vi "Periodic Tasks.vi"(8 "error in":errorcluster) -> ()   [LabVIEW 2017]
doc: "This VI runs in parallel to other tasks. It can contain as many user-defined periodic loops as you need. These can carry out PID or other sorts of timed response."
uses:
  elevator_control.ctl
  Intake_control.ctl
  <vilib>/Rock Robotics/WPI/ThirdParty/Phoenix-LabVIEW/Motor Controller/Controls/CTRE_Phoenix_MotorControl_ControlMode.ctl
  <vilib>/Rock Robotics/WPI/DriverStation/WPI_DriverStationRobotMode2.ctl
  <vilib>/Rock Robotics/WPI/Solenoid/WPI_SolenoidValue.ctl
  LabVIEW_is_Under_Control.lib/Util/Toggle/Change Detect.vi
  LabVIEW_is_Under_Control.lib/Util/Toggle/Change Detect Boolean.vi
  Robot Global Data.vi
  <vilib>/Rock Robotics/Network Tables/NT Write Boolean.vi
  <vilib>/Rock Robotics/Network Tables/NT Write String.vi
  <vilib>/Rock Robotics/Network Tables/NT Write Number.vi
  <vilib>/Rock Robotics/Network Tables/NT Read Boolean.vi
  <vilib>/Rock Robotics/WPI/Solenoid/WPI_SolenoidSetEnum.vi
panel:
  in  "Drive_proportional":dbl=0.8
  in  "Switch Height":dbl=40.0
  in  "Scoring Lower":dbl=55.0
  in  "Scale_Auto":dbl=-0.2
  in  "Switch_Auto":dbl=-0.4
  in  "Score Scale":dbl=-0.3
  in  "Exchange_Auto":dbl=40.0
  in  "Holding? Time":dbl=500.0 format="%#_13g"
  out "Elevador Encoder":dbl
  out "Yaw":dbl=-56.89
  in  "Exchange_Teleop":dbl=4.0
  in  "ScoringHigh":dbl=83.0
  in  "Scoring Low":dbl=67.0
  in  "Enable squared":bool
  in  "Score Switch":dbl=-1.0
  in  "Segurando":dbl=0.3
  in  "Expelir":dbl=-0.3
  in  "Coletar":dbl=0.7
  # "Para alterar:"
  # "Intake"
  # "Drivetrain"
  # "Elevador"
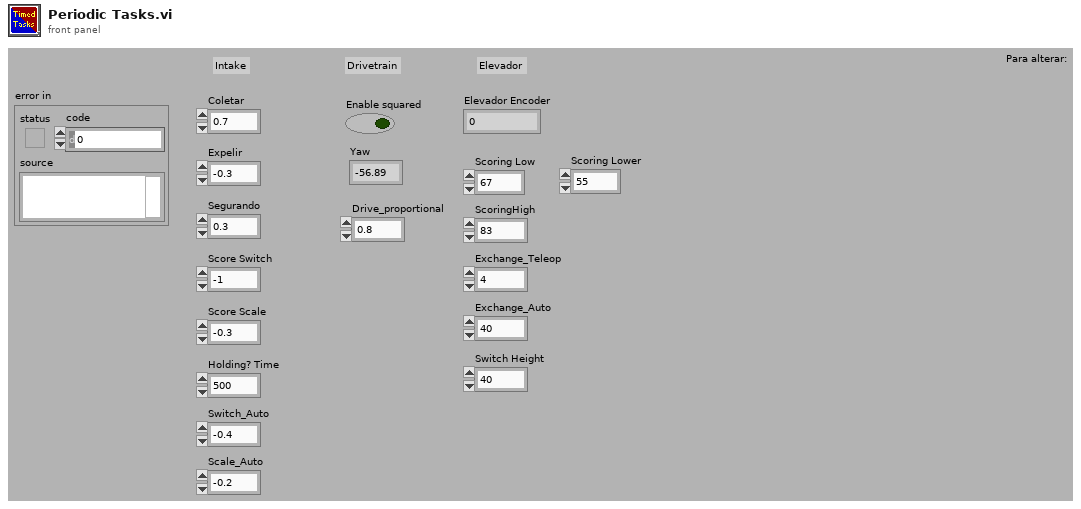
[diagram p1: front panel]
types:
  T1 = typedef "Intake_control.ctl" = enum16{"Repouso", "Coletando", "Segurando", "Score"}
  T2 = typedef "elevator_control.ctl" = enum16{"Resting", "Scoring Low", "Scoring Higher", "Exchange", "Scoring Lower", "Switch"}
  T3 = typedef "WPI_SwitchDevRef.ctl" = cluster{"DevStatus":errorcluster, "DIO Channel":T4, "CntIndex":T5, "Normally Closed":bool}
  T4 = typedef "FPGA_DIOChannel.ctl" = enum8{"DIO 0", "DIO 1", "DIO 2", "DIO 3", "DIO 4", "DIO 5", "DIO 6", "DIO 7", "DIO 8", "DIO 9", "DIO MXP 0", "DIO MXP 1", "DIO MXP 2", "DIO MXP 3", "DIO MXP 4", "DIO MXP 5", "DIO MXP 6", "DIO MXP 7", "DIO MXP 8", "DIO MXP 9", "DIO MXP 10", "DIO MXP 11", "DIO MXP 12", "DIO MXP 13", "DIO MXP 14", "DIO MXP 15", "SPI Port CS1", "SPI Port CS2", "SPI Port CS3", "SPI Port MISO", "SPI Port MOSI", "Invalid"}
  T5 = typedef "FPGA_CounterCtrSystemIndex.ctl" = enum8{"Ctr 0", "Ctr 1", "Ctr 2", "Ctr 3", "Ctr 4", "Ctr 5", "Ctr 6", "Ctr 7", "Invalid"}
  T6 = typedef "WPI_EncoderDevRef.ctl" = cluster{"DevStatus":errorcluster, "EncoderIndex":T7, "CounterIndex":T5, "DistancePerCount":dbl, "Decoding Type":T8}
  T7 = typedef "FPGA_EncoderIdx.ctl" = enum8{"Enc 0", "Enc 1", "Enc 2", "Enc 3", "Enc 4", "Enc 5", "Enc 6", "Enc 7", "Invalid"}
  T8 = typedef "WPI_EncoderType.ctl" = enum16{"1x", "2x", "4x"}
  T9 = typedef "WPI_SolenoidDevRef.ctl" = cluster{"DevStatus":errorcluster, "Pneumatics Control Module":u8, "Forward Solenoid Channel":T10, "Reverse Solenoid Channel":T10}
  T10 = typedef "WPI_SolenoidChannel.ctl" = enum8{"Solenoid 0", "Solenoid 1", "Solenoid 2", "Solenoid 3", "Solenoid 4", "Solenoid 5", "Solenoid 6", "Solenoid 7", "Invalid"}
  T11 = typedef "WPI_MotorControlDeviceRef.ctl" = cluster{"DeviceStatus":errorcluster, "Type":T12, "PWM":cluster{"PWM Channel":T13, "DeadBand":T14}, "CAN":cluster{"Device Number":u8, "SetOutput VI Ref":variant, "GetOutput VI Ref":variant, "Enable VI Ref":variant, "Disable VI Ref":variant, "Data":variant}, "Invert":bool, "DIO PWM":cluster{"PWM \"Enable\" Channel":T13, "DIOChannel":T4, "PWM Rate":dbl}}
  T12 = typedef "WPI_MotorControlType.ctl" = enum16{"PWM", "CAN", "DIO PWM"}
  T13 = typedef "FPGA_DIOPWMChannel.ctl" = enum8{"PWM 0", "PWM 1", "PWM 2", "PWM 3", "PWM 4", "PWM 5", "PWM 6", "PWM 7", "PWM 8", "PWM 9", "PWM MXP 0", "PWM MXP 1", "PWM MXP 2", "PWM MXP 3", "PWM MXP 4", "PWM MXP 5", "PWM MXP 6", "PWM MXP 7", "PWM MXP 8", "PWM MXP 9", "Invalid"}
  T14 = typedef "WPI_PWMDeadband.ctl" = cluster{"Name":string, "maxPositivePwm":i32, "minPositivePwm":i32, "centerPwm":i32, "maxNegativePwm":i32, "minNegativePwm":i32, "angularRange":u16}
  T15 = typedef "WPI_SolenoidValue.ctl" = enum16{"Off", "On", "Forward", "Reverse"}
  T16 = typedef "WPI_DriverStationRobotMode2.ctl" = enum16{"Autonomous Disabled", "Autonomous Enabled", "Teleop Disabled", "Teleop Enabled", "Disconnected", "Finish", "Test Disabled", "Test Enabled", "Emergency Stopped"}
  T17 = cluster{"Yaw":dbl, "Roll":dbl, "Pitch":dbl, "Heading":dbl, "Fused Heading":dbl}
  T18 = typedef "Button Cluster.ctl" = cluster{"Buttons[0]":bool, "Buttons[1]":bool, "Buttons[2]":bool, "Buttons[3]":bool, "Buttons[4]":bool, "Buttons[5]":bool, "Buttons[6]":bool, "Buttons[7]":bool, "Buttons[8]":bool, "Buttons[9]":bool}
  T19 = typedef "CTRE_Phoenix_MotorControl_ControlMode.ctl" = u16
  T20 = typedef "Axes Cluster.ctl" = cluster{"Axes[0]":dbl, "Axes[1]":dbl, "Axes[2]":dbl, "Axes[3]":dbl, "Axes[4]":dbl, "Axes[5]":dbl, "Axes[6]":dbl, "Axes[7]":dbl, "Axes[8]":dbl}
  T21 = typedef "D-Pad.ctl" = cluster{"Top":bool, "Bottom":bool, "None":bool, "Right":bool, "Left":bool}
  T22 = cluster{"proportional gain (Kc)":dbl, "integral time (Ti, min)":dbl, "derivative time (Td, min)":dbl}
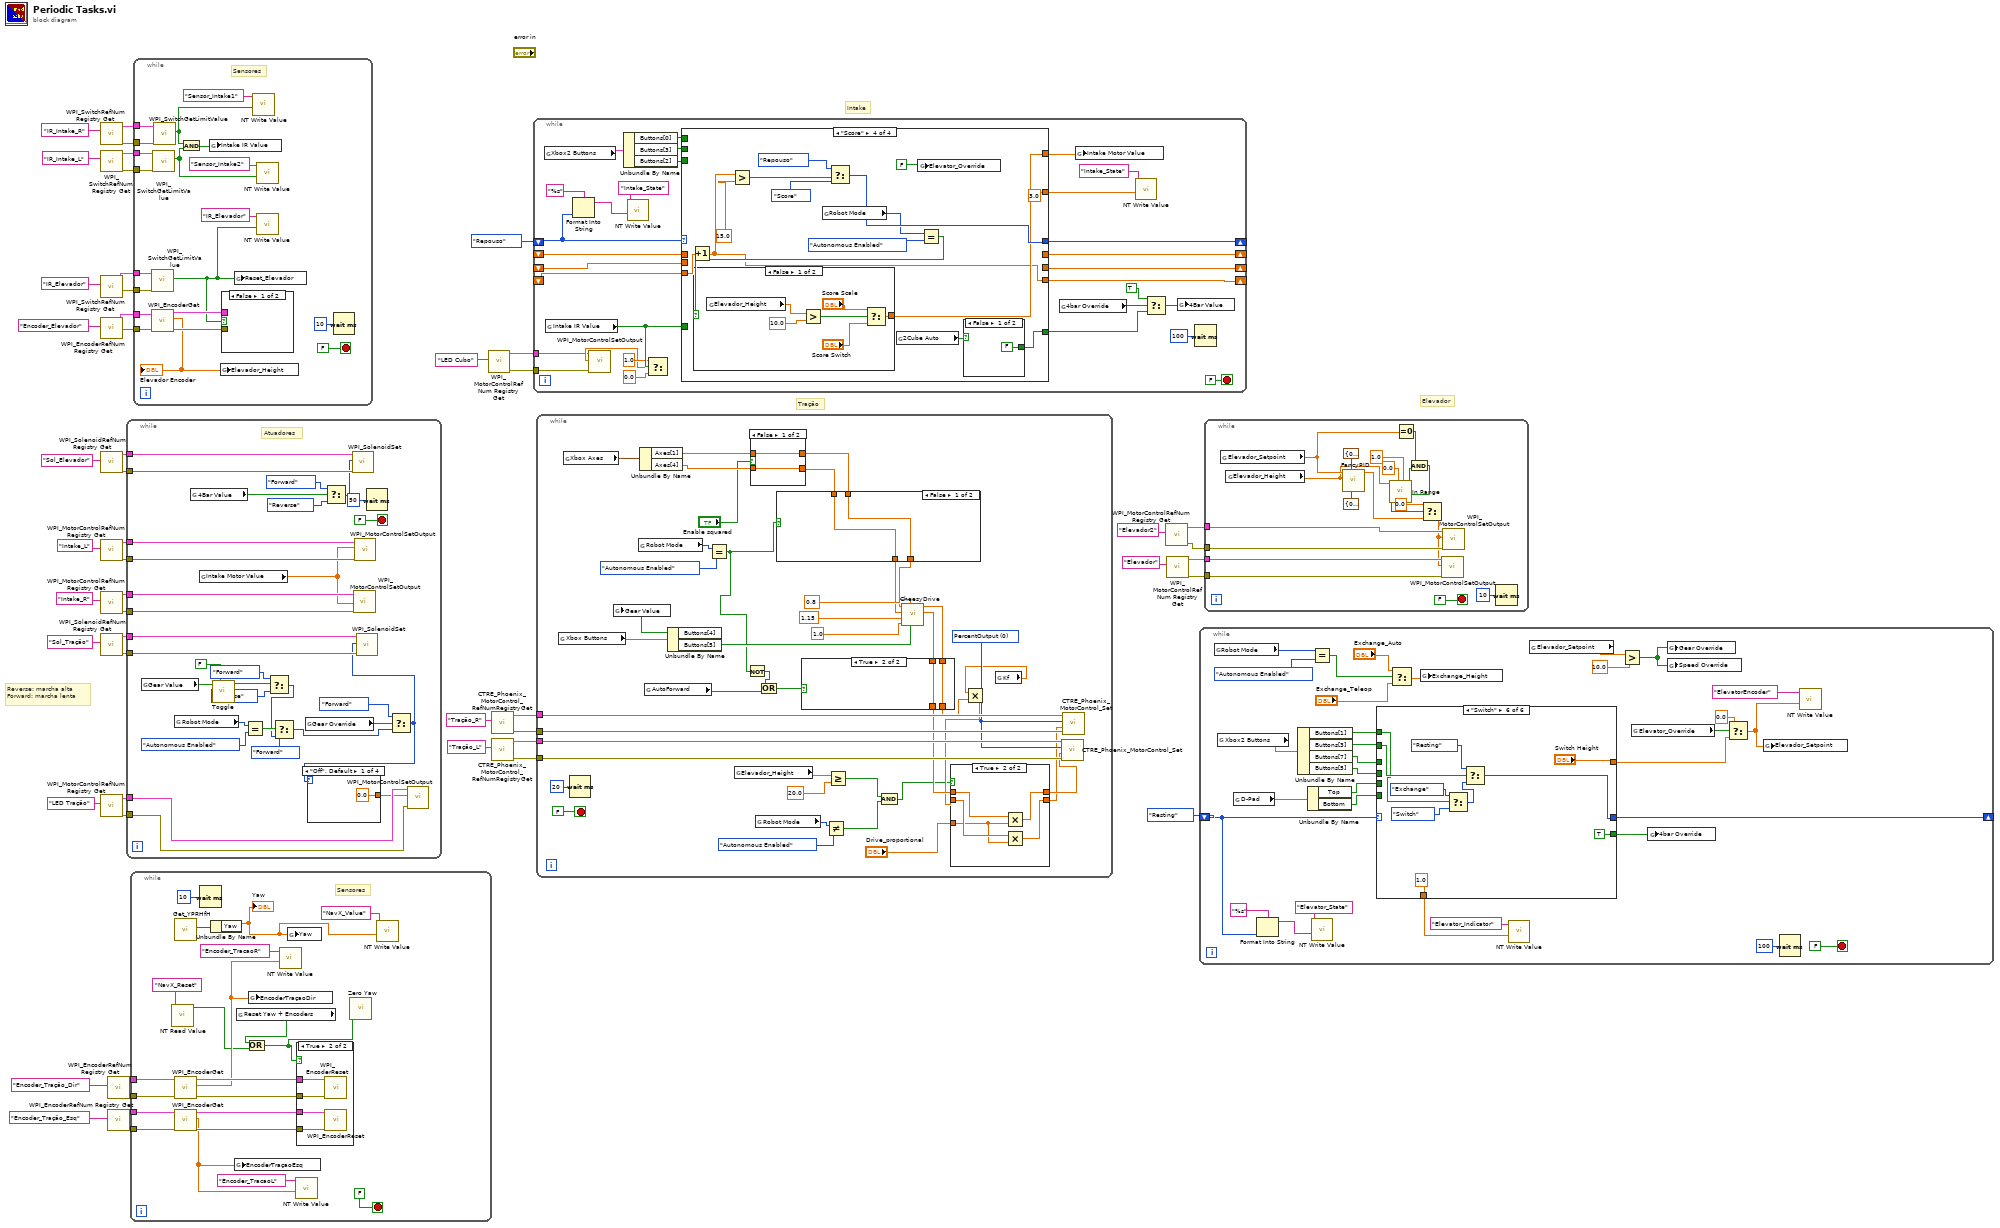
[diagram p0: block diagram]
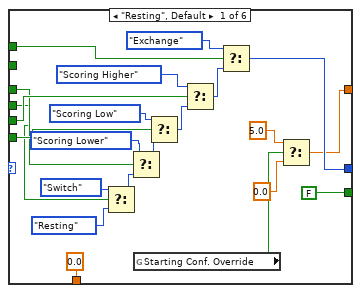
[diagram p3: hidden frame]
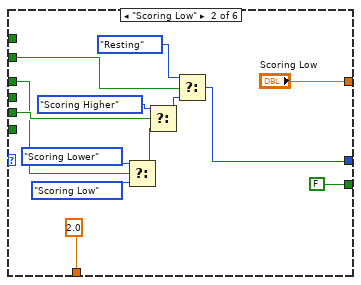
[diagram p4: hidden frame]
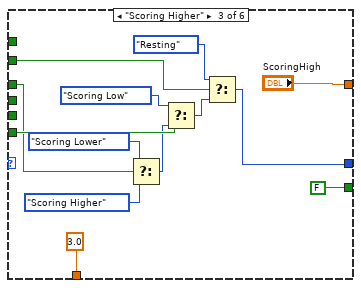
[diagram p5: hidden frame]
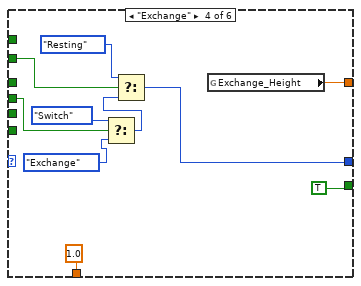
[diagram p6: hidden frame]
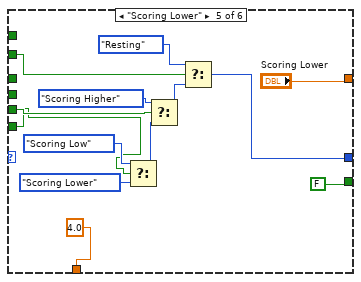
[diagram p7: hidden frame]
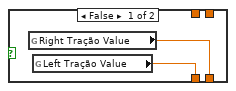
[diagram p9: hidden frame]
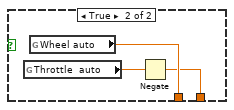
[diagram p10: hidden frame]
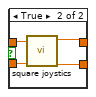
[diagram p11: hidden frame]
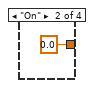
[diagram p12: hidden frame]
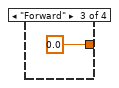
[diagram p13: hidden frame]
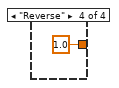
[diagram p14: hidden frame]
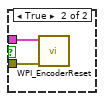
[diagram p15: hidden frame]
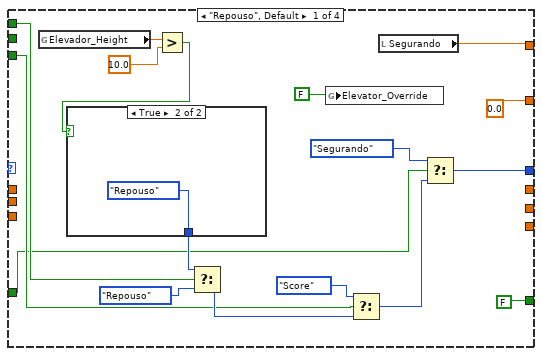
[diagram p16: hidden frame]
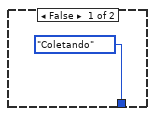
[diagram p17: hidden frame]
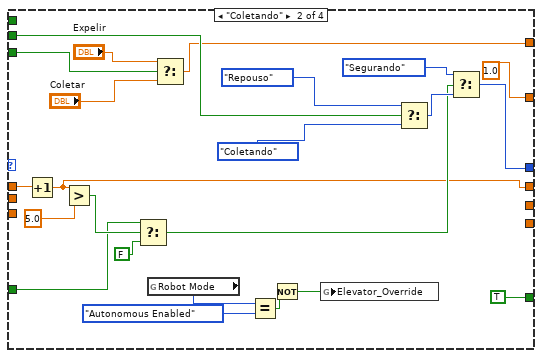
[diagram p18: hidden frame]
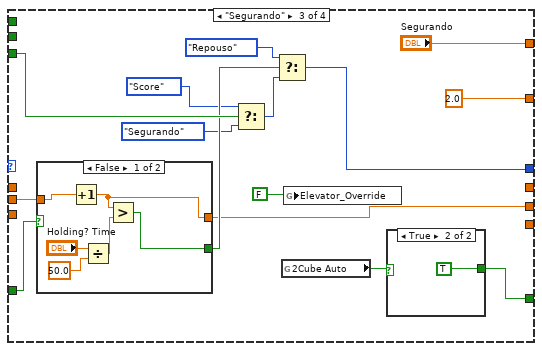
[diagram p19: hidden frame]
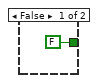
[diagram p20: hidden frame]
diagram:
  # "Reverse: marcha alta\nForward: marcha lenta"
  # "Elevador"
  # "Tração"
  # "Intake"
  n1 = call <vilib>:"WPI_SwitchRefNum Registry Get.vi"("refnum name"="IR_Intake_R") -> ("error out"=w46:errorcluster, "SwitchDevRef"=w45:T3)  [unwired: 9 in]
  n2 = call <vilib>:"WPI_SwitchRefNum Registry Get.vi"("refnum name"="IR_Intake_L") -> ("error out"=w48:errorcluster, "SwitchDevRef"=w47:T3)  [unwired: 9 in]
  n3 = call <vilib>:"WPI_SwitchRefNum Registry Get.vi"("refnum name"="IR_Elevador") -> ("error out"=w25:errorcluster, "SwitchDevRef"=w26:T3)  [unwired: 9 in]
  n4 = call <vilib>:"WPI_EncoderRefNum Registry Get.vi"("refnum name"="Encoder_Elevador") -> ("error out"=w21:errorcluster, "EncoderDevRef"=w22:T6)  [unwired: 9 in]
  n5 = call <vilib>:"WPI_SolenoidRefNum Registry Get.vi"("refnum name"="Sol_Elevador") -> ("error out"=w43:errorcluster, "SolenoidDevRef"=w42:T9)  [unwired: 9 in]
  n6 = call <vilib>:"WPI_MotorControlRefNum Registry Get.vi"("refnum name"="Intake_L") -> ("error out"=w41:errorcluster, "MotorControlDevRef"=w40:T11)  [unwired: 9 in]
  n7 = call <vilib>:"WPI_MotorControlRefNum Registry Get.vi"("refnum name"="Intake_R") -> ("error out"=w36:errorcluster, "MotorControlDevRef"=w37:T11)  [unwired: 9 in]
  n8 = call <vilib>:"WPI_SolenoidRefNum Registry Get.vi"("refnum name"="Sol_Tração") -> ("error out"=w33:errorcluster, "SolenoidDevRef"=w34:T9)  [unwired: 9 in]
  n9 = call <vilib>:"WPI_MotorControlRefNum Registry Get.vi"("refnum name"="LED Tração") -> ("error out"=w6:errorcluster, "MotorControlDevRef"=w5:T11)  [unwired: 9 in]
  n10 = call <vilib>:"WPI_EncoderRefNum Registry Get.vi"("refnum name"="Encoder_Tração_Dir") -> ("error out"=w14:errorcluster, "EncoderDevRef"=w15:T6)  [unwired: 9 in]
  n11 = call <vilib>:"WPI_EncoderRefNum Registry Get.vi"("refnum name"="Encoder_Tração_Esq") -> ("error out"=w13:errorcluster, "EncoderDevRef"=w12:T6)  [unwired: 9 in]
  n12 = while {
    tunnel: w43 -> [w82]
    tunnel: w42 -> [w81]
    tunnel: w41 -> [w76]
    tunnel: w40 -> [w75]
    tunnel: w37 -> [w74]
    tunnel: w36 -> [w73]
    tunnel: w34 -> [w67]
    tunnel: w33 -> [w66]
    tunnel: w6 -> [w53]
    tunnel: w5 -> [w52]
    stop <- FALSE stop-if-true
    # "Atuadores"
    n13 = global read "Robot Global Data.vi" "Gear Value"() -> (w65:bool)
    n14 = global read "Robot Global Data.vi" "Robot Mode"() -> (w63:T16)
    n15 = global read "Robot Global Data.vi" "4Bar Value"() -> (w77:bool)
    n16 = global read "Robot Global Data.vi" "Intake Motor Value"() -> (w72:dbl)
    n17 = call "Toggle.vi"("Initial Value"=FALSE, "In"=w65) -> ("Toggled"=w64:bool)  [unwired: 9 in]
    n18 = Equal?(x=w63, y=WPI_DriverStationRobotMode2."Autonomous Enabled") -> (x = y?=w61:bool)
    n19 = Select(t=WPI_SolenoidValue."Forward" ("Value"), s=w64, f=WPI_SolenoidValue."Reverse" ("Value")) -> (s? t:f=w59:T15)
    n20 = Select(t=WPI_SolenoidValue."Forward", s=w61, f=w59) -> (s? t:f=w55:T15)
    n21 = global read "Robot Global Data.vi" "Gear Override"() -> (w57:bool)
    n22 = Select(t=WPI_SolenoidValue."Forward" ("Value"), s=w77, f=WPI_SolenoidValue."Reverse" ("Value")) -> (s? t:f=w80:T15)
    n23 = call-poly <vilib>:"WPI_SolenoidSet.vi"("error in (no error)"=w82, "Value"=w80, "SolenoidDevRef"=w81) -> ()  [unwired: 7 in, 2 out]
    n24 = call <vilib>:"WPI_MotorControlSetOutput.vi"("error in (no error)"=w73, "Output"=w72, "MotorControlDevRef"=w74) -> ()  [unwired: 6 in, 3 out]
    n25 = call <vilib>:"WPI_MotorControlSetOutput.vi"("error in (no error)"=w76, "Output"=w72, "MotorControlDevRef"=w75) -> ()  [unwired: 6 in, 3 out]
    n26 = Wait (ms)(milliseconds to wait=u32 50) -> ()  [unwired: 1 out]
    n27 = Select(t=WPI_SolenoidValue."Forward", s=w57, f=w55) -> (s? t:f=w54:T15)
    n28 = case shown="\"Off\", Default" w54 {
      tunnel: [0.0 0.0 0.0 1.0] -> w51
      frame "Off", Default {
      }
      frame "On" {
      }
      frame "Forward" {
      }
      frame "Reverse" {
      }
    }
    n29 = call-poly <vilib>:"WPI_SolenoidSet.vi"("error in (no error)"=w66, "Value"=w54, "SolenoidDevRef"=w67) -> ()  [unwired: 7 in, 2 out]
    n30 = call <vilib>:"WPI_MotorControlSetOutput.vi"("error in (no error)"=w53, "Output"=w51, "MotorControlDevRef"=w52) -> ()  [unwired: 6 in, 3 out]
  }
  n31 = while {
    tunnel: w15 -> [w107]
    tunnel: w14 -> [w106]
    tunnel: w12 -> [w104]
    tunnel: w13 -> [w105]
    stop <- FALSE stop-if-true
    # "Sensores"
    n32 = call-poly <vilib>:"NT Read Value.vi"("Name"="NavX_Reset") -> ("Boolean"=w88:bool)  [unwired: 9 in, 1 out]
    n33 = call <vilib>:"Get_YPRHfH.vi"() -> ("YRPHfH"=w97:T17)  [unwired: 11 in]
    n34 = call <vilib>:"WPI_EncoderGet.vi"("error in (no error)"=w106, "EncoderDevRef"=w107) -> ("error out"=w100:errorcluster, "Distance"=w93:dbl, "EncoderDevRef"=w101:T6)  [unwired: 4 in, 3 out]
    n35 = call <vilib>:"WPI_EncoderGet.vi"("error in (no error)"=w105, "EncoderDevRef"=w104) -> ("error out"=w98:errorcluster, "Distance"=w95:dbl, "EncoderDevRef"=w99:T6)  [unwired: 4 in, 3 out]
    n36 = Wait (ms)(milliseconds to wait=u32 10) -> ()  [unwired: 1 out]
    n37 = Unbundle By Name(w97) -> ("Yaw"=w92:dbl)
    "Yaw" <- w92
    n38 = global write "Robot Global Data.vi" "EncoderTraçaoEsq"(w95) -> ()
    n39 = global read "Robot Global Data.vi" "Reset Yaw + Encoders"() -> (w89:bool)
    n40 = Or(x=w89, y=w88) -> (x .or. y?=w87:bool)
    n41 = global write "Robot Global Data.vi" "EncoderTraçaoDir"(w93) -> ()
    n42 = call-poly <vilib>:"NT Write Value.vi"("Numeric"=w93, "Name"="Encoder_TracaoR") -> ()  [unwired: 9 in, 1 out]
    n43 = global write "Robot Global Data.vi" "Yaw"(w92) -> ()
    n44 = call-poly <vilib>:"NT Write Value.vi"("Numeric"=w95, "Name"="Encoder_TracaoL") -> ()  [unwired: 9 in, 1 out]
    n45 = case shown="True" w87 {
      tunnel: w101 -> [_ w111]
      tunnel: w100 -> [_ w110]
      tunnel: w99 -> [_ w109]
      tunnel: w98 -> [_ w108]
      frame False {
      }
      frame True {
        n46 = call <vilib>:"WPI_EncoderReset.vi"("error in (no error)"=w110, "EncoderDevRef"=w111) -> ()  [unwired: 8 in, 2 out]
        n47 = call <vilib>:"WPI_EncoderReset.vi"("error in (no error)"=w108, "EncoderDevRef"=w109) -> ()  [unwired: 8 in, 2 out]
      }
    }
    n48 = call <vilib>:"Zero Yaw.vi"("Zero"=w87) -> ()  [unwired: 11 in]
    n49 = call-poly <vilib>:"NT Write Value.vi"("Numeric"=w92, "Name"="NavX_Value") -> ()  [unwired: 9 in, 1 out]
  }
  n50 = while {
    tunnel: w48 -> [w129]
    tunnel: w47 -> [w128]
    tunnel: w46 -> [w127]
    tunnel: w45 -> [w126]
    tunnel: w25 -> [w124]
    tunnel: w26 -> [w125]
    tunnel: w22 -> [w123]
    tunnel: w21 -> [w122]
    stop <- FALSE stop-if-true
    # "Sensores"
    n51 = call <vilib>:"WPI_SwitchGetLimitValue.vi"("error in (no error)"=w124, "SwitchDevRef"=w125) -> ("Switch Pressed"=w112:bool)  [unwired: 7 in, 2 out]
    n52 = call <vilib>:"WPI_EncoderGet.vi"("error in (no error)"=w122, "EncoderDevRef"=w123) -> ("error out"=w120:errorcluster, "Distance"=w119:dbl, "EncoderDevRef"=w121:T6)  [unwired: 4 in, 3 out]
    "Elevador Encoder" <- w119
    n53 = call <vilib>:"WPI_SwitchGetLimitValue.vi"("error in (no error)"=w129, "SwitchDevRef"=w128) -> ("Switch Pressed"=w116:bool)  [unwired: 7 in, 2 out]
    n54 = call <vilib>:"WPI_SwitchGetLimitValue.vi"("error in (no error)"=w127, "SwitchDevRef"=w126) -> ("Switch Pressed"=w114:bool)  [unwired: 7 in, 2 out]
    n55 = And(x=w114, y=w116) -> (x .and. y?=w115:bool)
    n56 = global write "Robot Global Data.vi" "Intake IR Value"(w115) -> ()
    n57 = global write "Robot Global Data.vi" "Elevador_Height"(w119) -> ()
    n58 = case shown="False" w112 {
      tunnel: w121 -> [_ w133]
      tunnel: w120 -> [_ w132]
      frame False {
      }
      frame True {
        n59 = call <vilib>:"WPI_EncoderReset.vi"("error in (no error)"=w132, "EncoderDevRef"=w133) -> ()  [unwired: 8 in, 2 out]
      }
    }
    n60 = global write "Robot Global Data.vi" "Reset_Elevador"(w112) -> ()
    n61 = call-poly <vilib>:"NT Write Value.vi"("Boolean"=w114, "Name"="Sensor_Intake1") -> ()  [unwired: 9 in, 1 out]
    n62 = call-poly <vilib>:"NT Write Value.vi"("Boolean"=w116, "Name"="Sensor_Intake2") -> ()  [unwired: 9 in, 1 out]
    n63 = call-poly <vilib>:"NT Write Value.vi"("Boolean"=w112, "Name"="IR_Elevador") -> ()  [unwired: 9 in, 1 out]
    n64 = Wait (ms)(milliseconds to wait=u32 10) -> ()  [unwired: 1 out]
  }
  n65 = call <vilib>:"WPI_MotorControlRefNum Registry Get.vi"("refnum name"="LED Cubo") -> ("error out"=w2:errorcluster, "MotorControlDevRef"=w3:T11)  [unwired: 9 in]
  n66 = call <vilib>:"CTRE_Phoenix_MotorControl_RefNumRegistryGet.vi"("refnum name"="Tração_R") -> ("error out"=w28:errorcluster, "PhoenixMotorControlDevRef"=w30:T11)  [unwired: 9 in]
  n67 = call <vilib>:"CTRE_Phoenix_MotorControl_RefNumRegistryGet.vi"("refnum name"="Tração_L") -> ("error out"=w27:errorcluster, "PhoenixMotorControlDevRef"=w29:T11)  [unwired: 9 in]
  n68 = while {
    shift-right: [w160] -> _
    shift-left: Intake_control."Repouso" -> [w144]
    shift-right: [w158] -> _
    shift-left: _ -> [w159]
    tunnel: w3 -> [w139]
    tunnel: w2 -> [w138]
    shift-right: [w136] -> _
    shift-left: _ -> [w137]
    shift-right: [w135] -> _
    shift-left: _ -> [w134]
    stop <- FALSE stop-if-true
    n69 = global read "Robot Global Data.vi" "Xbox2 Buttons"() -> (w161:T18)
    n70 = global read "Robot Global Data.vi" "Intake IR Value"() -> (w143:bool)
    n71 = Format Into String(format string="%s", w144) -> (resulting string=w146:string)  [unwired: 2 in, 1 out]
    n72 = Unbundle By Name(w161) -> ("Buttons[0]"=w154:bool, "Buttons[3]"=w156:bool, "Buttons[2]"=w155:bool)
    n73 = call-poly <vilib>:"NT Write Value.vi"("String"=w146, "Name"="Intake_State") -> ()  [unwired: 9 in, 1 out]
    n74 = Select(t=1.0, s=w143, f=0.0) -> (s? t:f=w140:dbl)
    n75 = call <vilib>:"WPI_MotorControlSetOutput.vi"("error in (no error)"=w138, "Output"=w140, "MotorControlDevRef"=w139) -> ()  [unwired: 6 in, 3 out]
    n76 = case shown="\"Score\"" w144 {
      tunnel: w154 -> [w180 _ _ _]
      tunnel: [w168 w203 w213 w243] -> w160
      tunnel: w156 -> [_ w205 _ _]
      tunnel: w155 -> [w177 w198 w220 _]
      tunnel: w159 -> [_ w195 _ _]
      tunnel: [_ w189 _ _] -> w158
      tunnel: [w175 w199 "Segurando" w240] -> w157
      tunnel: [FALSE TRUE w217 w242] -> w148
      tunnel: [0.0 1.0 2.0 3.0] -> w150
      tunnel: w143 -> [w170 w192 w216 _]
      tunnel: w137 -> [_ _ w210 _]
      tunnel: [_ _ w209 _] -> w136
      tunnel: [_ _ _ w234] -> w135
      tunnel: w134 -> [_ _ _ w233]
      frame "Repouso", Default {
        n77 = global read "Robot Global Data.vi" "Elevador_Height"() -> (w174:dbl)
        n78 = Greater?(x=w174, y=10.0) -> (0:w172:bool)
        n79 = case shown="True" w172 {
          tunnel: [Intake_control."Coletando" Intake_control."Repouso"] -> w171
          frame False {
          }
          frame True {
          }
        }
        n80 = Select(t=w171, s=w180, f=Intake_control."Repouso") -> (s? t:f=w178:T1)
        n81 = global write "Robot Global Data.vi" "Elevator_Override"(FALSE) -> ()
        n82 = Select(t=Intake_control."Score", s=w177, f=w178) -> (s? t:f=w169:T1)
        n83 = local read "Segurando"() -> (w175:dbl)
        n84 = Select(t=Intake_control."Segurando", s=w170, f=w169) -> (s? t:f=w168:T1)
      }
      frame "Coletando" {
        n85 = Increment(x=w195) -> (x+1=w189:dbl)
        n86 = Greater?(x=w189, y=5.0) -> (0:w193:bool)
        n87 = Select(t=w192, s=w193, f=FALSE) -> (s? t:f=w191:bool)
        n88 = global read "Robot Global Data.vi" "Robot Mode"() -> (w188:T16)
        n89 = Select(t="Expelir", s=w198, f="Coletar") -> (s? t:f=w199:dbl)
        n90 = Equal?(x=w188, y=WPI_DriverStationRobotMode2."Autonomous Enabled") -> (x = y?=w187:bool)
        n91 = Not(x=w187) -> (.not. x?=w185:bool)
        n92 = global write "Robot Global Data.vi" "Elevator_Override"(w185) -> ()
        n93 = Select(t=Intake_control."Repouso", s=w205, f=Intake_control."Coletando") -> (s? t:f=w200:T1)
        n94 = Select(t=Intake_control."Segurando", s=w191, f=w200) -> (s? t:f=w203:T1)
      }
      frame "Segurando" {
        n95 = case shown="False" w216 {
          tunnel: [w228 0.0] -> w209
          tunnel: [w227 FALSE] -> w214
          tunnel: w210 -> [w223 _]
          frame False {
            n96 = Increment(x=w223) -> (x+1=w228:dbl)
            n97 = Divide(x="Holding? Time", y=50.0) -> (x/y=w224:dbl)
            n98 = Greater?(x=w228, y=w224) -> (0:w227:bool)
          }
          frame True {
          }
        }
        n99 = Select(t=Intake_control."Score", s=w220, f=Intake_control."Segurando") -> (s? t:f=w215:T1)
        n100 = Select(t=Intake_control."Repouso", s=w214, f=w215) -> (s? t:f=w213:T1)
        n101 = global read "Robot Global Data.vi" "2Cube Auto"() -> (w211:bool)
        n102 = global write "Robot Global Data.vi" "Elevator_Override"(FALSE) -> ()
        n103 = case shown="True" w211 {
          tunnel: [FALSE TRUE] -> w217
          frame False {
          }
          frame True {
          }
        }
      }
      frame "Score" {
        n104 = Increment(x=w233) -> (x+1=w234:dbl)
        n105 = Greater?(x=w234, y=15.0) -> (0:w244:bool)
        n106 = global read "Robot Global Data.vi" "Robot Mode"() -> (w238:T16)
        n107 = Select(t=Intake_control."Repouso", s=w244, f=Intake_control."Score") -> (s? t:f=w243:T1)
        n108 = global read "Robot Global Data.vi" "2Cube Auto"() -> (w235:bool)
        n109 = global write "Robot Global Data.vi" "Elevator_Override"(FALSE) -> ()
        n110 = Equal?(x=w238, y=WPI_DriverStationRobotMode2."Autonomous Enabled") -> (x = y?=w236:bool)
        n111 = case shown="False" w236 {
          tunnel: [w250 w254] -> w240
          frame False {
            n112 = global read "Robot Global Data.vi" "Elevador_Height"() -> (w253:dbl)
            n113 = Greater?(x=w253, y=10.0) -> (0:w251:bool)
            n114 = Select(t="Score Scale", s=w251, f="Score Switch") -> (s? t:f=w250:dbl)
          }
          frame True {
            n115 = global read "Robot Global Data.vi" "Elevador_Height"() -> (w259:dbl)
            n116 = Greater?(x=w259, y=50.0) -> (0:w257:bool)
            n117 = Select(t="Scale_Auto", s=w257, f="Switch_Auto") -> (s? t:f=w254:dbl)
          }
        }
        n118 = case shown="False" w235 {
          tunnel: [FALSE TRUE] -> w242
          frame False {
          }
          frame True {
          }
        }
      }
    }
    n119 = global read "Robot Global Data.vi" "4bar Override"() -> (w153:bool)
    n120 = global write "Robot Global Data.vi" "Intake Motor Value"(w157) -> ()
    n121 = call-poly <vilib>:"NT Write Value.vi"("Numeric"=w150, "Name"="Intake_State") -> ()  [unwired: 9 in, 1 out]
    n122 = Select(t=TRUE, s=w153, f=w148) -> (s? t:f=w152:bool)
    n123 = global write "Robot Global Data.vi" "4Bar Value"(w152) -> ()
    n124 = Wait (ms)(milliseconds to wait=u32 100) -> ()  [unwired: 1 out]
  }
  n125 = while {
    tunnel: w30 -> [w293]
    tunnel: w29 -> [w292]
    tunnel: w28 -> [w291]
    tunnel: w27 -> [w290]
    stop <- FALSE stop-if-true
    w289 = T19 0 items=["PercentOutput"=0, "Position"=1, "Velocity"=2, "Current"=3, "Follower"=5, "MotionProfile"=6, "MotionMagic"=7, "MotionMagicArc"=8, "MotionProfileArc"=10, "Disabled"=15] ("Control Mode")
    n126 = global read "Robot Global Data.vi" "Xbox Buttons"() -> (w300:T18)
    n127 = global read "Robot Global Data.vi" "Xbox Axes"() -> (w302:T20)
    n128 = Wait (ms)(milliseconds to wait=u32 20) -> ()  [unwired: 1 out]
    n129 = global read "Robot Global Data.vi" "Robot Mode"() -> (w285:T16)
    n130 = Unbundle By Name(w302) -> ("Axes[1]"=w287:dbl, "Axes[4]"=w288:dbl)
    n131 = global read "Robot Global Data.vi" "AutoForward"() -> (w275:bool)
    n132 = Unbundle By Name(w300) -> ("Buttons[4]"=w298:bool, "Buttons[5]"=w299:bool)
    n133 = global write "Robot Global Data.vi" "Gear Value"(w298) -> ()
    n134 = Equal?(x=w285, y=WPI_DriverStationRobotMode2."Autonomous Enabled") -> (x = y?=w274:bool)
    n135 = global read "Robot Global Data.vi" "Elevador_Height"() -> (w266:dbl)
    n136 = Not(x=w274) -> (.not. x?=w277:bool)
    n137 = case shown="False" "Enable squared" {
      tunnel: w288 -> [w320 w324]
      tunnel: [w320 w323] -> w282
      tunnel: w287 -> [w319 w322]
      tunnel: [w319 w321] -> w283
      frame False {
      }
      frame True {
        n138 = call "square joystics.vi"("right joy"=w324, "left joy"=w322) -> ("Right Out"=w323:dbl, "Left Out"=w321:dbl)  [unwired: 8 in]
      }
    }
    n139 = global read "Robot Global Data.vi" "Robot Mode"() -> (w263:T16)
    n140 = Or(x=w277, y=w275) -> (x .or. y?=w276:bool)
    n141 = case shown="False" w274 {
      tunnel: [w314 w318] -> w278
      tunnel: [w315 w316] -> w279
      tunnel: w283 -> [w315 _]
      tunnel: w282 -> [w314 _]
      frame False {
      }
      frame True {
        n142 = global read "Robot Global Data.vi" "Throttle  auto"() -> (w317:dbl)
        n143 = global read "Robot Global Data.vi" "Wheel auto"() -> (w318:dbl)
        n144 = Negate(x=w317) -> (-x=w316:dbl)
      }
    }
    n145 = Not Equal?(x=w263, y=WPI_DriverStationRobotMode2."Autonomous Enabled") -> (x != y?=w260:bool)
    n146 = Greater Or Equal?(x=w266, y=20.0) -> (x >= y?=w262:bool)
    n147 = And(x=w262, y=w260) -> (x .and. y?=w261:bool)
    n148 = call "CheesyDrive.vi"("Quickturn"=w299, "WheelNonLinearity"=0.8, "negInertiaScalar"=1.0, "Sensitivty"=1.15, "Wheel"=w278, "Throttle"=w279) -> ("Right PWM"=w280:dbl, "Left PWM"=w281:dbl)  [unwired: 4 in]
    n149 = case shown="True" w276 {
      tunnel: [w310 w312] -> w273
      tunnel: w281 -> [_ w312]
      tunnel: [w311 w313] -> w271
      tunnel: w280 -> [_ w313]
      frame False {
        n150 = global read "Robot Global Data.vi" "Right Tração Value"() -> (w310:dbl)
        n151 = global read "Robot Global Data.vi" "Left Tração Value"() -> (w311:dbl)
      }
      frame True {
      }
    }
    n152 = global read "Robot Global Data.vi" "Kf"() -> (w272:dbl)
    n153 = Multiply(x=w272, y=w273) -> (x*y=w269:dbl)
    n154 = case shown="True" w261 {
      tunnel: w271 -> [w304 w309]
      tunnel: [w304 w308] -> w270
      tunnel: w269 -> [w303 w307]
      tunnel: [w303 w306] -> w268
      tunnel: "Drive_proportional" -> [_ w305]
      frame False {
      }
      frame True {
        n155 = Multiply(x=w309, y=w305) -> (x*y=w308:dbl)
        n156 = Multiply(x=w307, y=w305) -> (x*y=w306:dbl)
      }
    }
    n157 = call <vilib>:"CTRE_Phoenix_MotorControl_Set.vi"("error in (no error)"=w290, "Output"=w270, "Control Mode"=w289, "PhoenixMotorControlDevRef"=w292) -> ()  [unwired: 6 in, 2 out]
    n158 = call <vilib>:"CTRE_Phoenix_MotorControl_Set.vi"("error in (no error)"=w291, "Output"=w268, "Control Mode"=w289, "PhoenixMotorControlDevRef"=w293) -> ()  [unwired: 6 in, 2 out]
  }
  n159 = call <vilib>:"WPI_MotorControlRefNum Registry Get.vi"("refnum name"="Elevador2") -> ("error out"=w8:errorcluster, "MotorControlDevRef"=w9:T11)  [unwired: 9 in]
  n160 = call <vilib>:"WPI_MotorControlRefNum Registry Get.vi"("refnum name"="Elevador") -> ("error out"=w18:errorcluster, "MotorControlDevRef"=w19:T11)  [unwired: 9 in]
  n161 = while {
    shift-right: [w354] -> _
    shift-left: elevator_control."Resting" -> [w340]
    stop <- FALSE stop-if-true
    n162 = global read "Robot Global Data.vi" "Robot Mode"() -> (w339:T16)
    n163 = global read "Robot Global Data.vi" "Xbox2 Buttons"() -> (w349:T18)
    n164 = global read "Robot Global Data.vi" "D-Pad"() -> (w348:T21)
    n165 = Format Into String(format string="%s", w340) -> (resulting string=w342:string)  [unwired: 2 in, 1 out]
    n166 = Unbundle By Name(w349) -> ("Buttons[1]"=w347:bool, "Buttons[3]"=w346:bool, "Buttons[7]"=w326:bool, "Buttons[5]"=w325:bool)
    n167 = Unbundle By Name(w348) -> ("Top"=w345:bool, "Bottom"=w344:bool)
    n168 = Equal?(x=w339, y=WPI_DriverStationRobotMode2."Autonomous Enabled") -> (x = y?=w337:bool)
    n169 = call-poly <vilib>:"NT Write Value.vi"("String"=w342, "Name"="Elevator_State") -> ()  [unwired: 9 in, 1 out]
    n170 = case shown="\"Switch\"" w340 {
      tunnel: [w364 "Scoring Low" "ScoringHigh" w410 "Scoring Lower" "Switch Height"] -> w329
      tunnel: [w376 w389 w402 w414 w416 w434] -> w354
      tunnel: [FALSE FALSE FALSE TRUE FALSE TRUE] -> w353
      tunnel: [0.0 2.0 3.0 1.0 4.0 1.0] -> w351
      tunnel: w347 -> [w373 _ _ _ _ w429]
      tunnel: w346 -> [_ w385 w398 w411 w421 w433]
      tunnel: w345 -> [w372 w386 _ _ w420 _]
      tunnel: w344 -> [w371 _ w399 _ w417 _]
      tunnel: w326 -> [w362 w380 w393 _ _ _]
      tunnel: w325 -> [w357 _ _ w406 _ _]
      frame "Resting", Default {
        n171 = Select(t=elevator_control."Switch", s=w357, f=elevator_control."Resting") -> (s? t:f=w360:T2)
        n172 = Select(t=elevator_control."Scoring Lower", s=w362, f=w360) -> (s? t:f=w363:T2)
        n173 = global read "Robot Global Data.vi" "Starting Conf. Override"() -> (w369:bool)
        n174 = Select(t=elevator_control."Scoring Low", s=w371, f=w363) -> (s? t:f=w378:T2)
        n175 = Select(t=elevator_control."Scoring Higher", s=w372, f=w378) -> (s? t:f=w377:T2)
        n176 = Select(t=elevator_control."Exchange", s=w373, f=w377) -> (s? t:f=w376:T2)
        n177 = Select(t=5.0, s=w369, f=0.0 ("Exchange")) -> (s? t:f=w364:dbl)
      }
      frame "Scoring Low" {
        n178 = Select(t=elevator_control."Scoring Lower", s=w380, f=elevator_control."Scoring Low") -> (s? t:f=w382:T2)
        n179 = Select(t=elevator_control."Scoring Higher", s=w386, f=w382) -> (s? t:f=w390:T2)
        n180 = Select(t=elevator_control."Resting", s=w385, f=w390) -> (s? t:f=w389:T2)
      }
      frame "Scoring Higher" {
        n181 = Select(t=elevator_control."Scoring Lower", s=w393, f=elevator_control."Scoring Higher") -> (s? t:f=w395:T2)
        n182 = Select(t=elevator_control."Scoring Low", s=w399, f=w395) -> (s? t:f=w403:T2)
        n183 = Select(t=elevator_control."Resting", s=w398, f=w403) -> (s? t:f=w402:T2)
      }
      frame "Exchange" {
        n184 = Select(t=elevator_control."Switch", s=w406, f=elevator_control."Exchange") -> (s? t:f=w408:T2)
        n185 = Select(t=elevator_control."Resting", s=w411, f=w408) -> (s? t:f=w414:T2)
        n186 = global read "Robot Global Data.vi" "Exchange_Height"() -> (w410:dbl)
      }
      frame "Scoring Lower" {
        n187 = Select(t=elevator_control."Scoring Low", s=w417, f=elevator_control."Scoring Lower") -> (s? t:f=w424:T2)
        n188 = Select(t=elevator_control."Scoring Higher", s=w420, f=w424) -> (s? t:f=w427:T2)
        n189 = Select(t=elevator_control."Resting", s=w421, f=w427) -> (s? t:f=w416:T2)
      }
      frame "Switch" {
        n190 = Select(t=elevator_control."Exchange", s=w429, f=elevator_control."Switch") -> (s? t:f=w431:T2)
        n191 = Select(t=elevator_control."Resting", s=w433, f=w431) -> (s? t:f=w434:T2)
      }
    }
    n192 = Select(t="Exchange_Auto", s=w337, f="Exchange_Teleop") -> (s? t:f=w334:dbl)
    n193 = global write "Robot Global Data.vi" "Exchange_Height"(w334) -> ()
    n194 = call-poly <vilib>:"NT Write Value.vi"("Numeric"=w351, "Name"="Elevator_Indicator") -> ()  [unwired: 9 in, 1 out]
    n195 = global read "Robot Global Data.vi" "Elevador_Setpoint"() -> (w327:dbl)
    n196 = Greater?(x=w327, y=10.0) -> (0:w328:bool)
    n197 = global read "Robot Global Data.vi" "Elevator_Override"() -> (w332:bool)
    n198 = global write "Robot Global Data.vi" "4bar Override"(w353) -> ()
    n199 = global write "Robot Global Data.vi" "Gear Override"(w328) -> ()
    n200 = global write "Robot Global Data.vi" "Speed Override"(w328) -> ()
    n201 = Select(t=0.0, s=w332, f=w329) -> (s? t:f=w330:dbl)
    n202 = global write "Robot Global Data.vi" "Elevador_Setpoint"(w330) -> ()
    n203 = Wait (ms)(milliseconds to wait=u32 100) -> ()  [unwired: 1 out]
    n204 = call-poly <vilib>:"NT Write Value.vi"("Numeric"=w330, "Name"="ElevatorEncoder") -> ()  [unwired: 9 in, 1 out]
  }
  n205 = while {
    tunnel: w19 -> [w453]
    tunnel: w18 -> [w452]
    tunnel: w9 -> [w449]
    tunnel: w8 -> [w448]
    stop <- FALSE stop-if-true
    n206 = global read "Robot Global Data.vi" "Elevador_Setpoint"() -> (w447:dbl)
    n207 = global read "Robot Global Data.vi" "Elevador_Height"() -> (w440:dbl)
    n208 = call "FancyPID.vi"("Gains"=T22 {"proportional gain (Kc)"=0.095, "integral time (Ti, min)"=0.007, "derivative time (Td, min)"=0.0} ("Gains Elevador"), "Range"=cluster{"output high":dbl, "output low":dbl} {"output high"=0.95, "output low"=-0.25} ("Range Elevador"), "Process variable"=w440, "Setpoint"=w447) -> ("output"=w444:dbl)  [unwired: 7 in]
    n209 = call "In Range.vi"("Range"=1.0, "Setpoint"=0.0, "Value"=w440) -> ("in range?"=w441:bool)  [unwired: 8 in]
    n210 = Equal To 0?(x=w447) -> (x = 0?=w446:bool)
    n211 = And(x=w446, y=w441) -> (x .and. y?=w445:bool)
    n212 = Select(t=0.0, s=w445, f=w444) -> (s? t:f=w442:dbl)
    n213 = call <vilib>:"WPI_MotorControlSetOutput.vi"("error in (no error)"=w452, "Output"=w442, "MotorControlDevRef"=w453) -> ()  [unwired: 6 in, 3 out]
    n214 = call <vilib>:"WPI_MotorControlSetOutput.vi"("error in (no error)"=w448, "Output"=w442, "MotorControlDevRef"=w449) -> ()  [unwired: 6 in, 3 out]
    n215 = Wait (ms)(milliseconds to wait=u32 10) -> ()  [unwired: 1 out]
  }
